vi "Run important tasks.vi"(7 "pulses previous":dbl, 8 "error in (no error)":errorcluster, 9 "ControlQueue":refnum<queue>, 10 "divider":i8=10, 11 "DAQmxTaskContainer_General in":refnum<class "DAQmxTaksContainer_General.lvclass">) -> (0 "error out":errorcluster, 2 "pulses":dbl, 3 "DAQmxTaskContainer_General out":refnum<class "DAQmxTaksContainer_General.lvclass">)   [LabVIEW 2015, in "DAQmxTaskContainer.lvclass"]
uses:
  DAQmxTaskContainer/DAQmxTaskContainer.lvclass
  DAQmxTaksContainer_General.lvclass
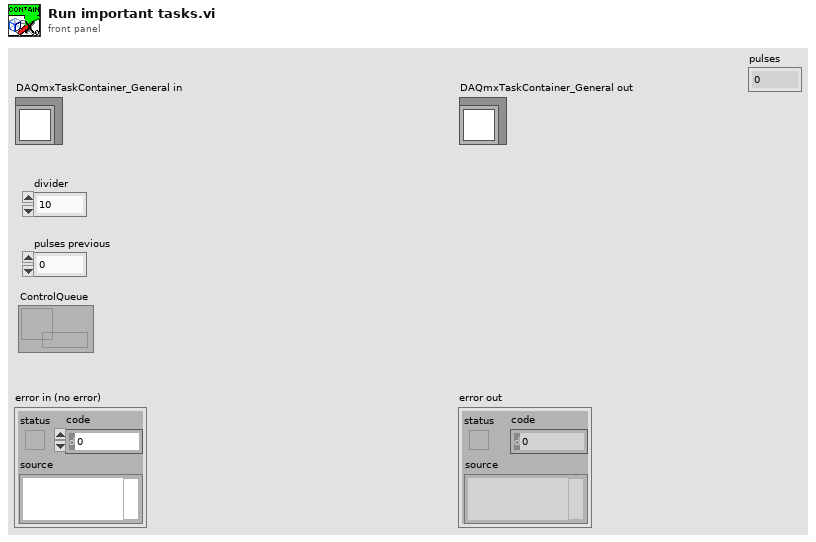
[diagram p1: front panel]
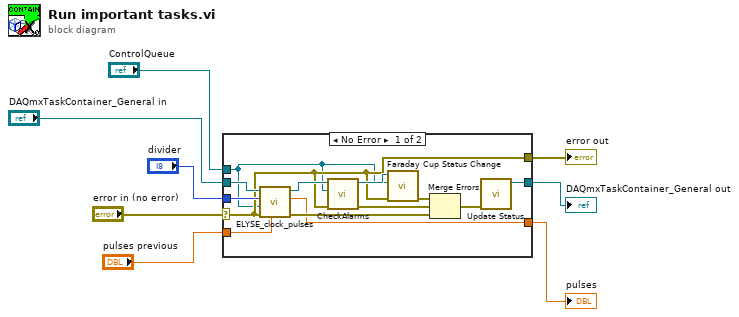
[diagram p0: block diagram]
diagram:
  n1 = case shown="No Error" "error in (no error)" {
    selector: "error in (no error)" -> [w13 w24]
    tunnel: [w13 w24] -> w7
    tunnel: [w16 w23] -> w5
    tunnel: "DAQmxTaskContainer_General in" -> [w17 w23]
    tunnel: "divider" -> [w15 _]
    tunnel: "ControlQueue" -> [w11 _]
    tunnel: "pulses previous" -> [w10 w22]
    tunnel: [w9 w22] -> w1
    frame No Error {
      n2 = call "ELYSE_clock_pulses.vi"("pulses previous"=w10, "error in (no error)"=w13, "ControlQueue"=w11, "divider"=w15, "DAQmxTaksContainer_General in"=w17) -> ("error out"=w20:errorcluster, "pulses"=w9:dbl, "DAQmxTaksContainer_General out"=w19:refnum<class "DAQmxTaksContainer_General.lvclass">)  [unwired: 4 in]
      n3 = call "CheckAlarms.vi"("error in (no error)"=w13, "ControlQueue"=w11, "DAQmxTaksContainer_General in"=w19) -> ("error out"=w21:errorcluster, "DAQmxTaksContainer_General out"=w14:refnum<class "DAQmxTaksContainer_General.lvclass">)  [unwired: 7 in]
      n4 = call-dynamic "Faraday Cup Status Change.vi"("error in (no error)"=w13, "ControlQueue"=w11, "DAQmxTaskContainer in"=w14) -> ("error out"=w12:errorcluster)  [unwired: 7 in, 1 out]
      n5 = Merge Errors(w12, w21, w20) -> (w18:errorcluster)
      n6 = call "Update Status.vi"("error in (no error)"=w18) -> ("DAQmxTaskContainer en sortie"=w16:refnum<class "DAQmxTaskContainer.lvclass">)  [unwired: 8 in, 2 out]
    }
    frame Error {
    }
  }
  "error out" <- w7
  "DAQmxTaskContainer_General out" <- w5
  "pulses" <- w1
